vi "TrajFilter.vi"(6 "AnkleTraj_Init":bool, 9 "Traj of Current Step":dbl[][](array[numeric])) -> (0 "AnkleTraj_Init dup":bool, 3 "AverageTraj":dbl[][](array[numeric]))   [LabVIEW 2016, in "ForceField.lvclass"]
uses:
  ForceField.lvclass
panel:
  in  "b":dbl[](array[numeric])=[1.0, 0.0, 0.1716]
  in  "a":dbl[](array[numeric])=[0.2929, 0.5858, 0.2929]
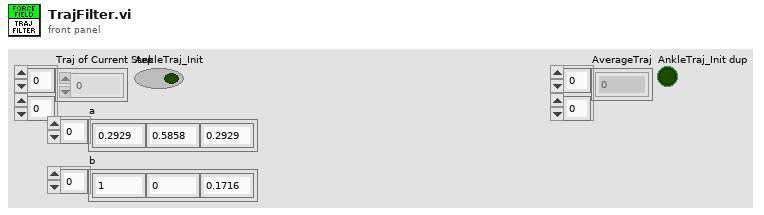
[diagram p1: front panel]
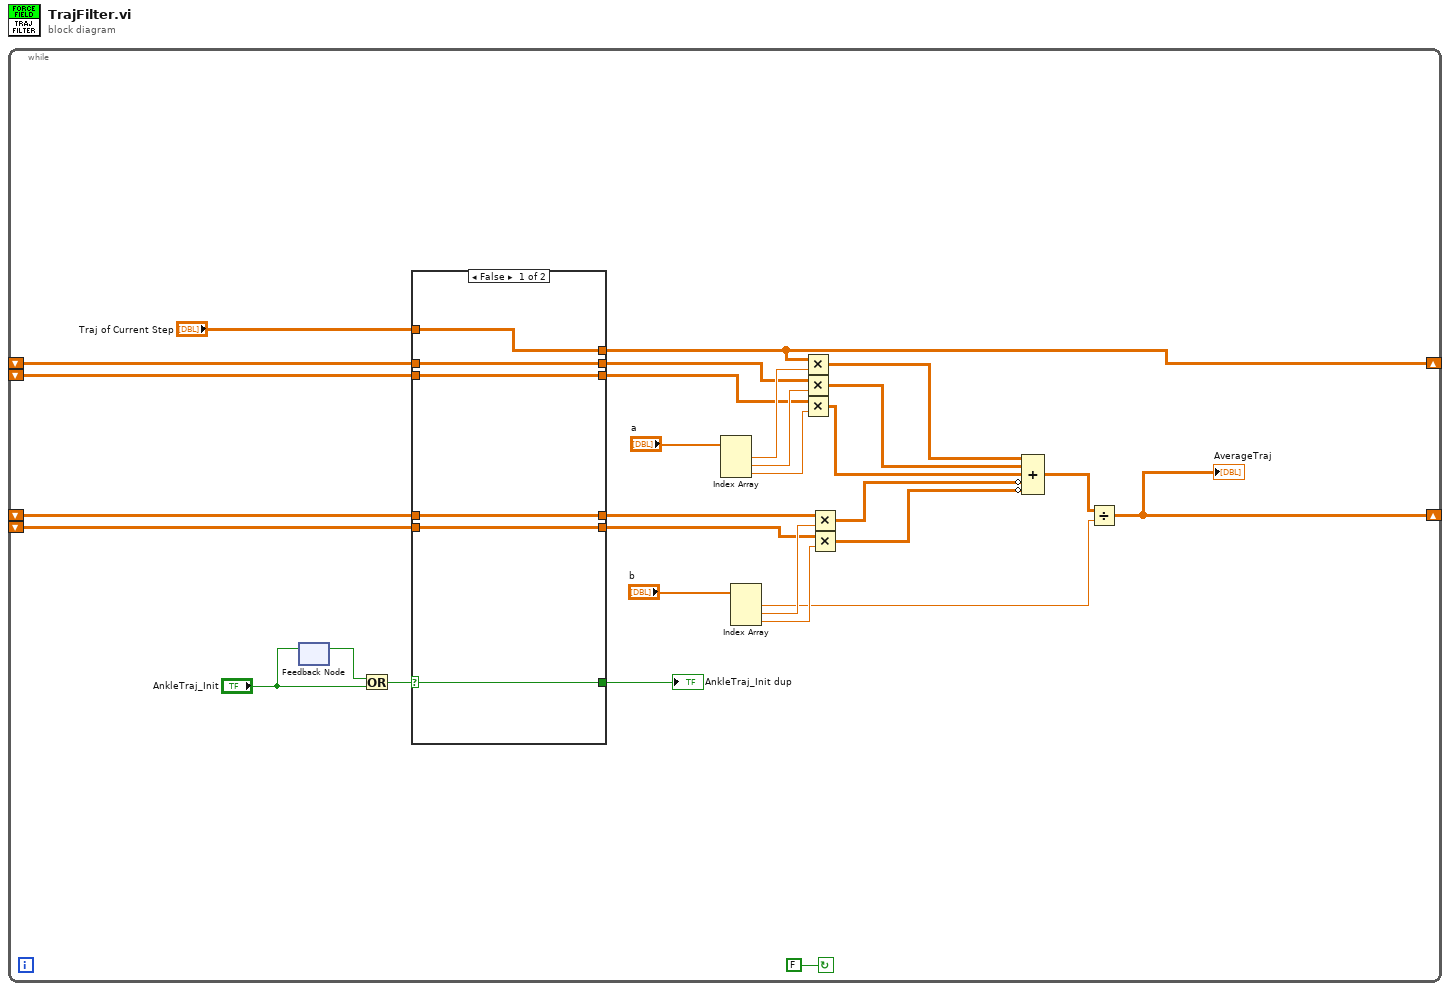
[diagram p0: block diagram]
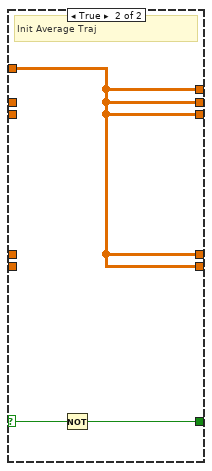
[diagram p2: hidden frame]
diagram:
  n1 = while {
    shift-right: [w28] -> _
    shift-left: _ -> [w13]
    shift-left: _ -> [w10]
    shift-right: [w15] -> _
    shift-left: _ -> [w8]
    shift-left: _ -> [w6]
    stop <- FALSE continue-if-true
    n2 = feedback-in #1("AnkleTraj_Init") -> ()
    n3 = feedback #1() -> (w2:bool)  [unwired: 1 in]
    n4 = Or(x=w2, y="AnkleTraj_Init") -> (x .or. y?=w3:bool)
    n5 = case shown="False" w3 {
      selector: w3 -> [w32 w38]
      tunnel: [w31 w39] -> w28
      tunnel: w13 -> [w35 _]
      tunnel: [w35 w39] -> w12
      tunnel: "Traj of Current Step" -> [w31 w39]
      tunnel: w10 -> [w36 _]
      tunnel: [w36 w39] -> w9
      tunnel: w8 -> [w34 _]
      tunnel: [w34 w39] -> w7
      tunnel: w6 -> [w33 _]
      tunnel: [w33 w39] -> w5
      tunnel: [w32 w37] -> w4
      frame False {
      }
      frame True {
        # "Init Average Traj"
        n6 = Not(x=w38) -> (.not. x?=w37:bool)
      }
    }
    "AnkleTraj_Init dup" <- w4
    n7 = Index Array(array="a") -> (element #1=w27:dbl, element #2=w26:dbl, element #3=w25:dbl)  [unwired: 3 in]
    n8 = Index Array(array="b") -> (element #1=w14:dbl, element #2=w20:dbl, element #3=w19:dbl)  [unwired: 3 in]
    n9 = Multiply(x=w28, y=w27) -> (x*y=w24:dbl[][])
    n10 = Multiply(x=w12, y=w26) -> (x*y=w23:dbl[][])
    n11 = Multiply(x=w9, y=w25) -> (x*y=w22:dbl[][])
    n12 = Multiply(x=w7, y=w20) -> (x*y=w18:dbl[][])
    n13 = Multiply(x=w5, y=w19) -> (x*y=w17:dbl[][])
    n14 = Compound Arithmetic op=ADD(w24, w23, w22, invert w18, invert w17) -> (w16:dbl[][])
    n15 = Divide(x=w16, y=w14) -> (x/y=w15:dbl[][])
    "AverageTraj" <- w15
  }
